vi "LængdeMåler.vi"() -> ()   [LabVIEW 2022 SP3]
uses:
  <vilib>/express/express arith-compare/Formula/XNode/ExpressFormulaBlockNode.xnode
panel:
  out "OK?":bool
  out "Over?":string
  in  "Max":dbl
  out "Numeric 3":dbl
  in  "Tid":dbl
  in  "Speed":dbl
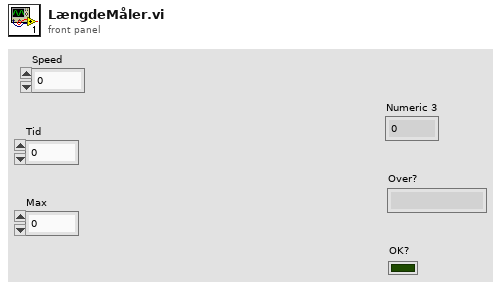
[diagram p1: front panel]
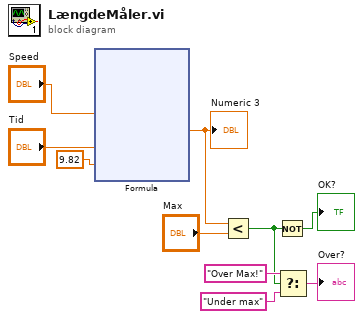
[diagram p0: block diagram]
diagram:
  n1 = xnode "Formula"("u"="Speed", "t"="Tid", "a"=9.82 ("t")) -> ("Result"=w5:dbl)  [unwired: 1 in, 1 out]
  "Numeric 3" <- w5
  n2 = Less?(x=w5, y="Max") -> (x < y?=w2:bool)
  n3 = Not(x=w2) -> (.not. x?=→"OK?":bool)
  n4 = Select(t="Over Max!", s=w2, f="Under max") -> (s? t:f=→"Over?":string)
